vi "SAOMM-CameraParamsFixer.vi"(0 "PRAMMS-COMM IN":refnum<visa-resource-name>="Hp\u0000\u0002", 1 "Signature":u32=1886544237, 2 "Active Refnum":refnum<vi>, 3 "ACK Refnum":refnum<vi>, 5 "ValueUpdated":u16(ring) items=["Binning", "ROISize", "ROIXoffset", "ROIYoffset", "RefPixX", "RefPixY"], 7 "Old value":dbl, 9 "New Value":dbl, 11 "Error IN":errorcluster, 12 "Offset":cluster{"ROIYOffset":u16, "ROIXOffset":u16}, 13 "Size":cluster{"ROIWidth":u16, "ROIHeight":u16}, 14 "RefPix":cluster{"X":dbl, "Y":dbl}) -> (4 "PRAMMS-COMM OUT":refnum<visa-resource-name>, 15 "Error OUT":errorcluster)   [LabVIEW 2011]
panel:
  in  "MessageType":cluster{string[], u32[]}={["emtError", "emtAreYouThere", "emtAcknowledgment", "emtGetClientType", "emtClientType", "emtGetImageExposureTime", "emtSetImageExposureTime", "emtImageExposureTime", "emtGetOptimalExposureTime", "emtSetOptimalExposureTime", "emtOptimalExposureTime", "emtGetImageEMGain", "emtSetImageEMGain", "emtImageEMGain", "emtGetFPGACtrl", "emtSetFPGACtrl", "emtFPGACtrl", "emtGetImageWidth", "emtSetImageWidth", "emtImageWidth", "emtGetImageHeight", "emtSetImageHeight", "emtImageHeight", "emtGetImageBinning", "emtSetImageBinning", "emtImageBinning", "emtGetImageDisplayFrameRate", "emtSetImageDisplayFrameRate", "emtImageDisplayFrameRate", "emtGetROIWidth", "emtSetROIWidth", "emtROIWidth", "emtGetROIHeight", "emtSetROIHeight", "emtROIHeight", "emtGetROIXOffset", "emtSetROIXOffset", "emtROIXOffset", "emtGetROIYOffset", "emtSetROIYOffset", "emtROIYOffset", "emtStartAcquisition", "mtStopAcquisition", "emtAcquisitionStarted", "emtAcquisitionStopped", "emtGetFalconImage", "emtFalconImage"], [1, 2, 3, 4, 5, 1001, 1101, 1201, 1002, 1102, 1202, 1003, 1103, 1203, 1004, 1104, 1204, 1005, 1105, 1205, 1006, 1106, 1206, 1007, 1107, 1207, 1008, 1108, 1208, 1009, 1109, 1209, 1010, 1110, 1210, 1011, 1111, 1211, 1012, 1112, 1212, 1130, 1131, 1150, 1151, 1070, 1270]}
  in  "Binning":u16(ring) items=["1 x 1"=1, "2 x 2"=2, "4 x 4"=4, "5 x 5"=5]
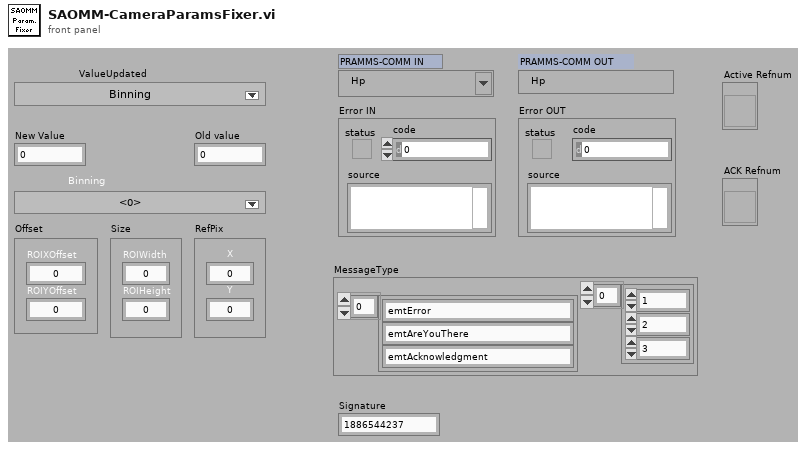
[diagram p1: front panel]
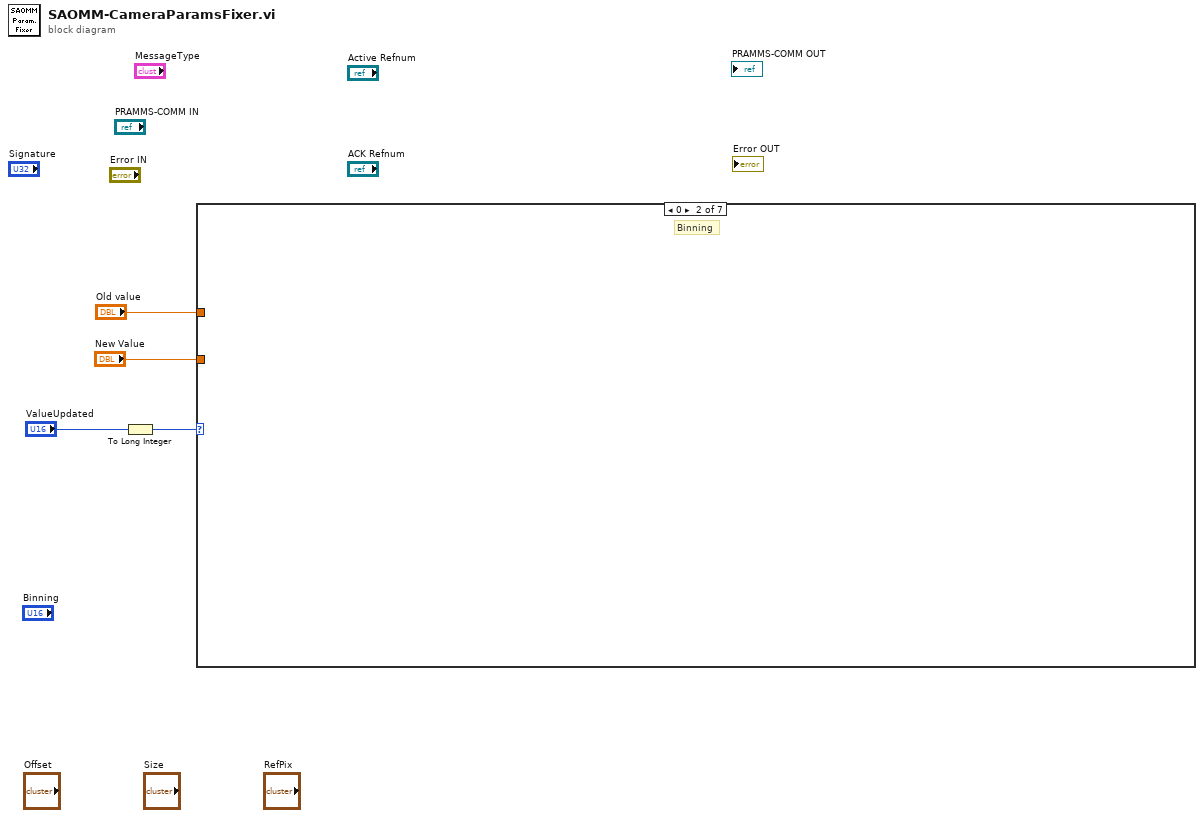
[diagram p0: block diagram]
diagram:
  n1 = To Long Integer(number="ValueUpdated") -> (32bit integer=w3:i32)
  n2 = case shown="0" w3 {
    tunnel: "Old value" -> [_ _ _ _ _ _ _]
    tunnel: "New Value" -> [_ _ _ _ _ _ _]
    frame -1, Default {
    }
    frame 0 {
      # "Binning"
    }
    frame 1 {
      # "ROI Size"
    }
    frame 2 {
      # "ROIXOffset"
    }
    frame 3 {
      # "ROIYOffset"
    }
    frame 4 {
      # "RefPixelX"
    }
    frame 5 {
      # "RefPixY"
    }
  }
